vi "DegToRad.vi"(1 "fi in degrees":i32) -> (0 "fi in radians":dbl)   [LabVIEW 2020]
doc: "Degrees (0, infinity) to radians (0, 2pi)"
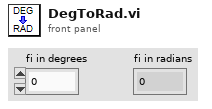
[diagram p1: front panel]
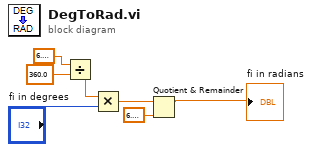
[diagram p0: block diagram]
diagram:
  n1 = Divide(x=6.283185307179586, y=360.0) -> (x/y=w4:dbl)
  n2 = Multiply(x=w4, y="fi in degrees") -> (x*y=w5:dbl)
  n3 = Quotient & Remainder(x=w5, y=6.283185307179586) -> (x-y*floor(x/y)=→"fi in radians":dbl)  [unwired: 1 out]
